vi "s-lab第5章 簇数据1-6.vi"() -> ()   [LabVIEW 2013]
panel:
  out "字符数组":string[](array[string])=["h", "j", "k", "l"]
  out "数值数组":i32[](array[numeric])=[0, 2, 4, 6, 8]
  out "合并后的 簇数组":cluster{i32, string}[](array[cluster])
  out "簇数组":T1(array[cluster])
  in  "簇 7":cluster{"数值":dbl, "布尔":bool, "字符串":string}
  in  "簇 6":cluster{"数值":dbl, "布尔":bool, "字符串":string}
  out "字符串输出 2":string
  out "布尔 3":bool
  out "数值输出 2":dbl
  out "旋钮输出 2":dbl
  in  "簇 5":T2 {"旋钮" scale=0.0..10.0}
  in  "替换字符串":string
  in  "替换数值":dbl
  out "簇 4":cluster{"数值":dbl, "字符串":string}
  in  "簇 3":cluster{"数值":dbl, "字符串":string}
  out "字符串输出":string
  out "布尔 2":bool
  out "数值输出":dbl
  out "旋钮输出":dbl
  in  "簇 2":T2 {"旋钮" scale=0.0..10.0}
  in  "字符串":string
  in  "布尔":bool
  in  "旋钮":dbl(knob) scale=0.0..10.0
  out "簇":cluster{"数值":dbl, "布尔":bool, "字符串":string}
  # "例 1"
  # "例 2"
  # "例 3"
  # "例 4"
  # "例 5"
  # "注意：此处创建的簇数组，只能在“创建簇数组函数”的输出端右键，然后选择“创建-显示控件”。\n      如果自己创建一个数组，然后添加簇，在然后添加簇元素，创建成的显示控件是无法使用的。"
  # "例 6"
  # "注意：此处创建的簇数组，由“索引与捆绑簇数组函数”的输出端右键，然后选择“创建-显示控件”创建。\n      新的簇数组按照原数组中最短一个数组建立"
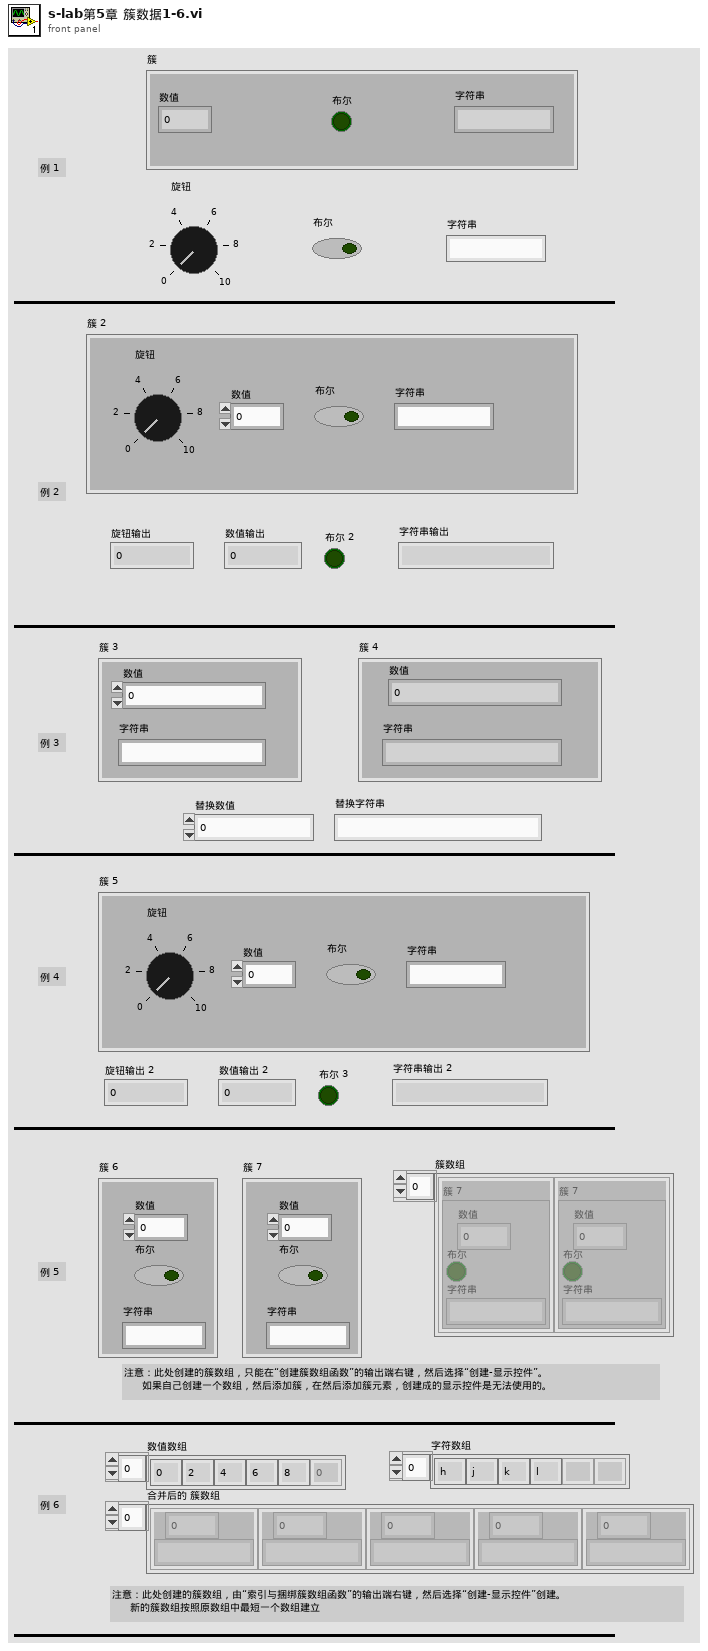
[diagram p1: front panel]
types:
  T1 = cluster{"簇 7":cluster{"数值":dbl, "布尔":bool, "字符串":string}}[]
  T2 = cluster{"旋钮":dbl, "数值":dbl, "布尔":bool, "字符串":string}
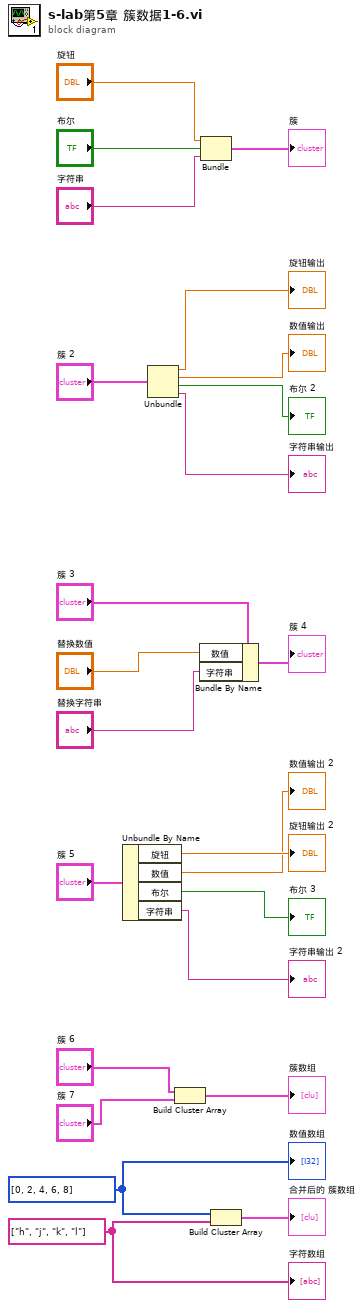
[diagram p0: block diagram]
diagram:
  w2 = string[] ["h", "j", "k", "l"]
  w3 = i32[] [0, 2, 4, 6, 8]
  n1 = Unbundle By Name("簇 5") -> ("旋钮"=→"旋钮输出 2":dbl, "数值"=→"数值输出 2":dbl, "布尔"=→"布尔 3":bool, "字符串"=→"字符串输出 2":string)
  n2 = Unbundle("簇 2") -> ("旋钮"=→"旋钮输出":dbl, "数值"=→"数值输出":dbl, "布尔"=→"布尔 2":bool, "字符串"=→"字符串输出":string)
  n3 = Build Cluster Array("簇 6", "簇 7") -> (→"簇数组":T1)
  n4 = Bundle By Name(cluster="簇 3", "数值"="替换数值", "字符串"="替换字符串") -> (→"簇 4":cluster{"数值":dbl, "字符串":string})
  n5 = Bundle("旋钮"="旋钮", "布尔"="布尔", "字符串"="字符串") -> (→"簇":cluster{"旋钮":dbl, "布尔":bool, "字符串":string})  [unwired: 1 in]
  n6 = Build Cluster Array(w3, w2) -> (→"合并后的 簇数组":cluster{i32, string}[])
  "数值数组" <- w3
  "字符数组" <- w2
